vi "IQvalidate.vi"(0 "Ystart":dbl, 1 "Xstart":dbl, 2 "Depth Map":dbl[][](array[numeric]), 5 "baseline, mm":sgl, 7 "ppx":sgl, 9 "ppy":sgl, 11 "fy":sgl, 12 "fx":sgl) -> (3 "rms %":dbl, 4 "AngleY":dbl, 6 "rms error value, mm":dbl, 8 "AngleX":dbl, 10 "mean Z Value, mm":dbl, 13 "Fill factor (%) \n(new)":dbl=100.0, 14 "PointCloud":cluster{"x":dbl, "y":dbl, "z":dbl}[](array[cluster]), 15 "Subpixel, pix":dbl)   [LabVIEW 2017, in "libRealSense3.lvlib"]
uses:
  libRealSense3.lvlib
panel:
  out "error out":errorcluster
  in  "error in (no error)":errorcluster
  # "RS3 IQvalidate"
  # "(C) Intel Corp. 2020,  AGJ"
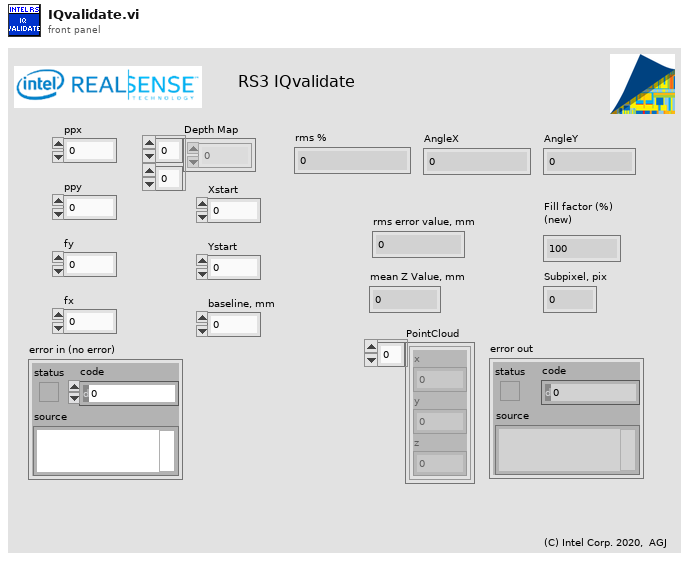
[diagram p1: front panel]
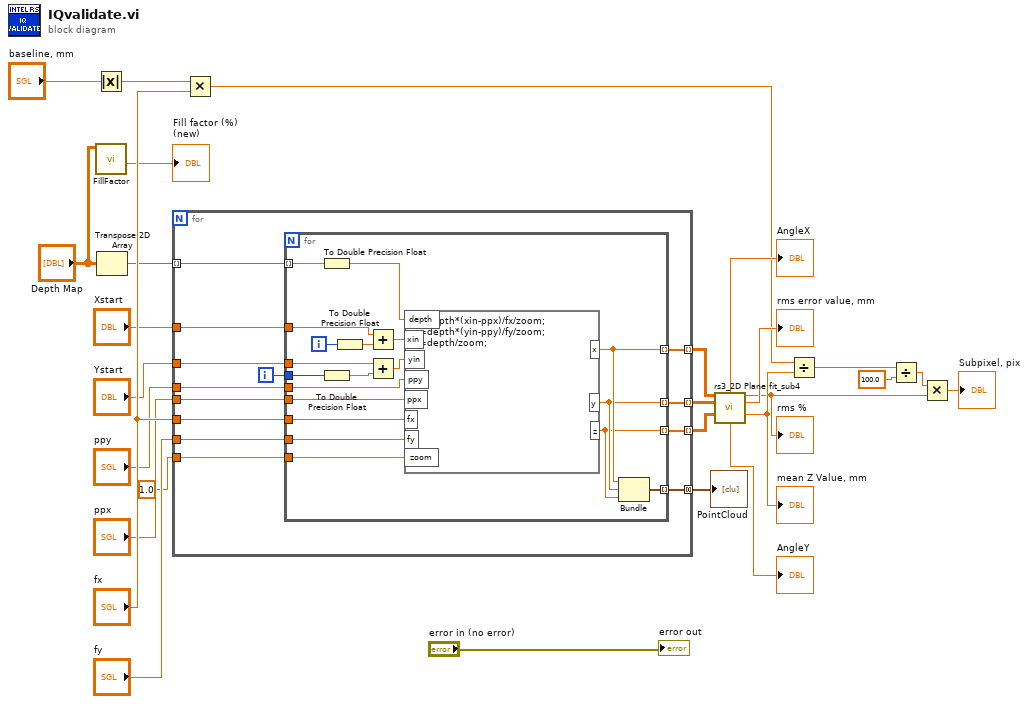
[diagram p0: block diagram]
diagram:
  n1 = Absolute Value(x="baseline, mm") -> (abs(x)=w13:sgl)
  n2 = call "FillFactor.vi"("Depth Output"="Depth Map") -> ("Fill factor (%)"=→"Fill factor (%) \n(new)":dbl)  [unwired: 8 in, 2 out]
  n3 = Transpose 2D Array(2D array="Depth Map") -> (transposed array=w5:dbl[][])
  n4 = for {
    tunnel: w5 -> [w40] mode=indexing
    tunnel: [w39] -> w4 mode=concatenating
    tunnel: [w37] -> w14 mode=indexing
    tunnel: [w36] -> w15 mode=indexing
    tunnel: [w35] -> w16 mode=indexing
    tunnel: "Xstart" -> [w34]
    tunnel: "Ystart" -> [w33]
    tunnel: 1.0 ("Scale (10=100um)") -> [w32]
    tunnel: "fx" -> [w31]
    tunnel: "fy" -> [w30]
    tunnel: "ppx" -> [w29]
    tunnel: "ppy" -> [w28]
    i -> [w38]
    n5 = for {
      tunnel: w40 -> [w59] mode=indexing
      tunnel: w38 -> [w58]
      tunnel: [w57] -> w39 mode=indexing
      tunnel: [w55] -> w37 mode=indexing
      tunnel: [w54] -> w36 mode=indexing
      tunnel: [w53] -> w35 mode=indexing
      tunnel: w34 -> [w51]
      tunnel: w33 -> [w47]
      tunnel: w32 -> [w45]
      tunnel: w31 -> [w44]
      tunnel: w30 -> [w43]
      tunnel: w29 -> [w42]
      tunnel: w28 -> [w41]
      i -> [w56]
      n6 = To Double Precision Float(number=w59) -> (double precision float=w52:dbl)
      n7 = To Double Precision Float(number=w58) -> (double precision float=w48:dbl)
      n8 = To Double Precision Float(number=w56) -> (double precision float=w49:dbl)
      n9 = Add(x=w51, y=w49) -> (x+y=w50:dbl)
      n10 = Add(x=w47, y=w48) -> (x+y=w46:dbl)
      n11 = formula code="x=depth*(xin-ppx)/fx/zoom;\ny=depth*(yin-ppy)/fy/zoom;\nz=depth/zoom;"("ppy"=w41, "ppx"=w42, "fx"=w44, "fy"=w43, "xin"=w50, "yin"=w46, "depth"=w52, "zoom"=w45) -> ("x"=w55:dbl, "y"=w54:dbl, "z"=w53:dbl)
      n12 = Bundle("x"=w55, "y"=w54, "z"=w53) -> (w57:cluster{"x":dbl, "y":dbl, "z":dbl})  [unwired: 1 in]
    }
  }
  "PointCloud" <- w4
  n13 = Multiply(x=w13, y="fx") -> (x*y=w6:sgl)
  n14 = call "rs3_2D Plane fit_sub4.vi"("Pointcloud X"=w14, "Pointcloud Y"=w15, "Pointcloud Z"=w16) -> ("AngleX"=→"AngleX":dbl, "rms %"=w12:dbl, "rms error value"=→"rms error value, mm":dbl, "mean Z Value"=w17:dbl, "AngleY"=→"AngleY":dbl)  [unwired: 3 in, 5 out]
  "mean Z Value, mm" <- w17
  "rms %" <- w12
  n15 = Divide(x=w6, y=w17) -> (x/y=w7:dbl)
  n16 = Divide(x=w7, y=100.0) -> (x/y=w9:dbl)
  n17 = Multiply(x=w9, y=w12) -> (x*y=→"Subpixel, pix":dbl)
  "error out" <- "error in (no error)"
